vi "eMIC_calibration.vi"(11 "eMIC data in":T1) -> (3 "eMIC data out":T1)   [LabVIEW 2018, in "Application.lvlib"]
uses:
  Application.lvlib
  eMIC response.ctl
panel:
  out "error out":errorcluster
  in  "error in (no error)":errorcluster
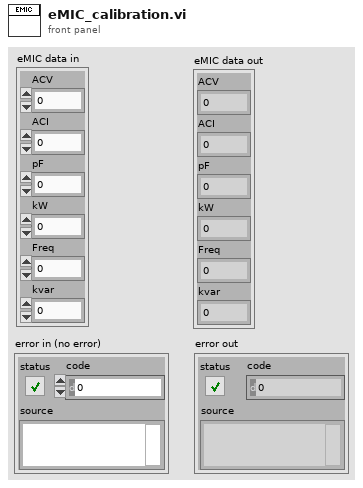
[diagram p1: front panel]
types:
  T1 = typedef "Application.lvlib/eMIC response.ctl" = cluster{"ACV":dbl, "ACI":dbl, "pF":dbl, "kW":dbl, "Freq":dbl, "kvar":dbl}
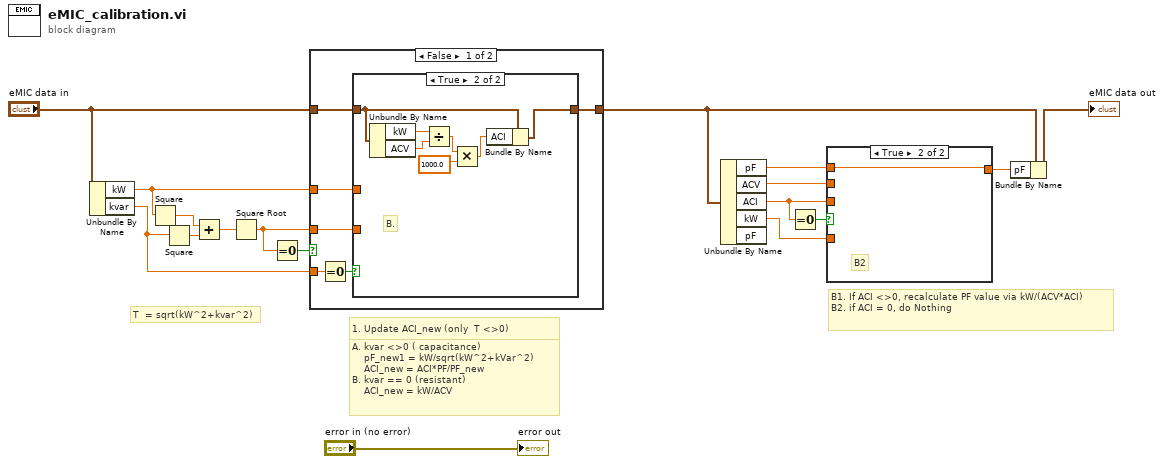
[diagram p0: block diagram]
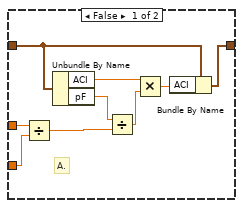
[diagram p2: hidden frame]
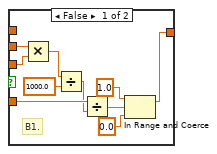
[diagram p4: hidden frame]
diagram:
  # "T  = sqrt(kW^2+kvar^2)"
  # "1. Update ACI_new (only  T <>0)"
  # "A. kvar <>0 ( capacitance)\n    pF_new1 = kW/sqrt(kW^2+kVar^2)\n    ACI_new = ACI*PF/PF_new\nB. kvar == 0 (resistant)\n    ACI_new = kW/ACV"
  # "B1. If ACI <>0, recalculate PF value via kW/(ACV*ACI)\nB2. if ACI = 0, do Nothing"
  n1 = Unbundle By Name("eMIC data in") -> ("kW"=w7:dbl, "kvar"=w3:dbl)
  n2 = Square(x=w7) -> (x^2=w6:dbl)
  n3 = Square(x=w3) -> (x^2=w5:dbl)
  n4 = Add(x=w6, y=w5) -> (x+y=w4:dbl)
  n5 = Square Root(x=w4) -> (sqrt(x)=w1:dbl)
  n6 = Equal To 0?(x=w1) -> (x = 0?=w2:bool)
  n7 = case shown="False" w2 {
    tunnel: w1 -> [w23 _]
    tunnel: w7 -> [w22 _]
    tunnel: "eMIC data in" -> [w21 w40]
    tunnel: [w20 w40] -> w9
    tunnel: w3 -> [w19 _]
    frame False {
      n8 = Equal To 0?(x=w19) -> (x = 0?=w18:bool)
      n9 = case shown="True" w18 {
        tunnel: w23 -> [w32 _]
        tunnel: w22 -> [w31 _]
        tunnel: w21 -> [w30 w37]
        tunnel: [w29 w36] -> w20
        frame False {
          # "A."
          n10 = Divide(x=w31, y=w32) -> (x/y=w28:dbl)
          n11 = Unbundle By Name(w30) -> ("ACI"=w25:dbl, "pF"=w27:dbl)
          n12 = Divide(x=w27, y=w28) -> (x/y=w24:dbl)
          n13 = Multiply(x=w25, y=w24) -> (x*y=w26:dbl)
          n14 = Bundle By Name(cluster=w30, "ACI"=w26) -> (w29:T1)
        }
        frame True {
          # "B."
          n15 = Unbundle By Name(w37) -> ("kW"=w39:dbl, "ACV"=w38:dbl)
          n16 = Divide(x=w39, y=w38) -> (x/y=w34:dbl)
          n17 = Multiply(x=w34, y=1000.0) -> (x*y=w33:dbl)
          n18 = Bundle By Name(cluster=w37, "ACI"=w33) -> (w36:T1)
        }
      }
    }
    frame True {
      # "T == 0\nDo nothing!"
    }
  }
  n19 = Unbundle By Name(w9) -> ("pF"=w11:dbl, "ACV"=w13:dbl, "ACI"=w15:dbl, "kW"=w14:dbl)  [unwired: 1 out]
  n20 = Equal To 0?(x=w15) -> (x = 0?=w16:bool)
  n21 = case shown="True" w16 {
    tunnel: w13 -> [w50 _]
    tunnel: w14 -> [w47 _]
    tunnel: w15 -> [w45 _]
    tunnel: w11 -> [_ w51]
    tunnel: [w41 w51] -> w10
    frame False {
      # "B1."
      n22 = Multiply(x=w50, y=w45) -> (x*y=w49:dbl)
      n23 = Divide(x=w49, y=1000.0) -> (x/y=w46:dbl)
      n24 = Divide(x=w47, y=w46) -> (x/y=w43:dbl)
      n25 = In Range and Coerce(upper limit=1.0, x=w43, lower limit=0.0) -> (coerced(x)=w41:dbl)  [unwired: 1 out]
    }
    frame True {
      # "B2"
    }
  }
  n26 = Bundle By Name(cluster=w9, "pF"=w10) -> (→"eMIC data out":T1)
  "error out" <- "error in (no error)"
